vi "Excersie 4.vi"() -> ()   [LabVIEW 2017]
panel:
  out "Indicator 3":bool
  out "Indicator 4":string
  out "Indicator 2":dbl
  out "Indicator 1":dbl
  in  "Input 4":string
  in  "Input 3":bool
  in  "Input 2":dbl
  in  "Input 1":dbl
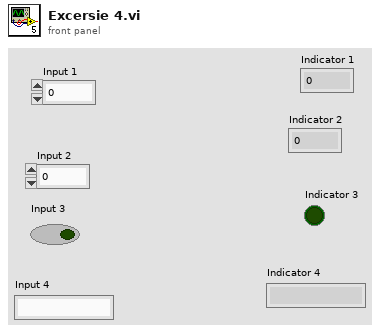
[diagram p1: front panel]
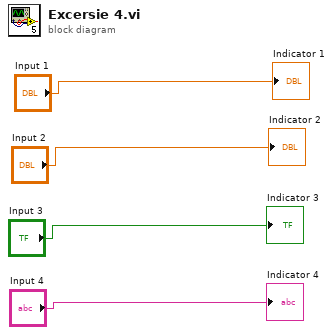
[diagram p0: block diagram]
diagram:
  "Indicator 1" <- "Input 1"
  "Indicator 2" <- "Input 2"
  "Indicator 4" <- "Input 4"
  "Indicator 3" <- "Input 3"
